vi "Date time format to text sortable.vi"(8 "error in (no error)":errorcluster, 11 "Date time string":string) -> (0 "error out":errorcluster, 3 "New date time string":string)   [LabVIEW 2013]
panel:
  out "PM?":bool
  out "minute":string
  out "hour":string
  out "year":string
  out "day":string="Day"
  out "month":string
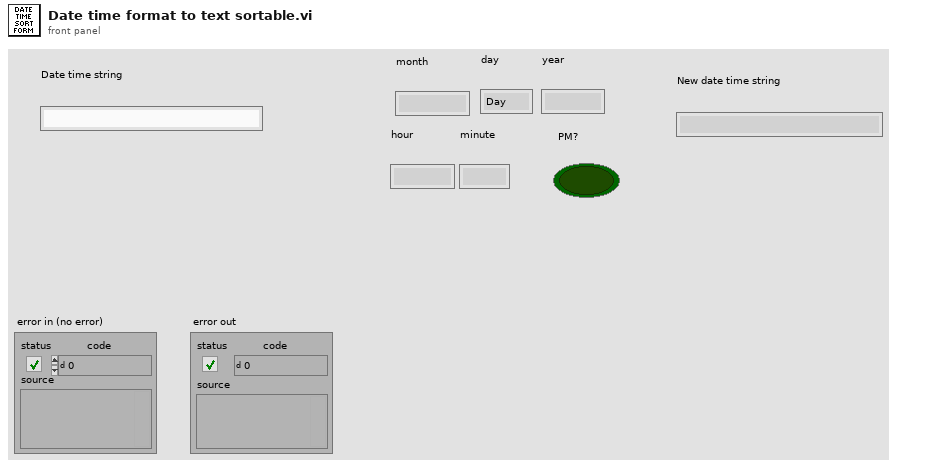
[diagram p1: front panel]
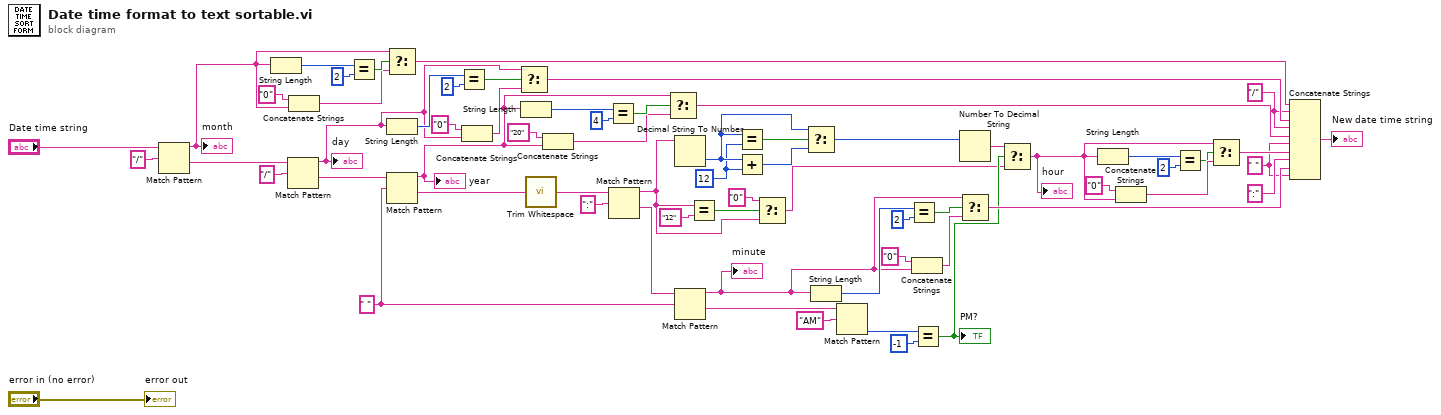
[diagram p0: block diagram]
diagram:
  w10 = 12 ("y")
  w15 = " " ("string")
  w37 = "/" ("string")
  w59 = " " ("regular expression")
  n1 = Match Pattern(string="Date time string", regular expression="/") -> (before substring=w48:string, after substring=w64:string)  [unwired: 1 in, 2 out]
  "month" <- w48
  n2 = String Length(string=w48) -> (length=w51:i32)
  n3 = Match Pattern(string=w64, regular expression="/") -> (before substring=w39:string, after substring=w62:string)  [unwired: 1 in, 2 out]
  "day" <- w39
  n4 = Concatenate Strings("0" ("string"), w48) -> (w46:string)
  n5 = Equal?(x=w51, y=2) -> (x = y?=w49:bool)
  n6 = Select(t=w48, s=w49, f=w46) -> (s? t:f=w45:string)
  n7 = String Length(string=w39) -> (length=w40:i32)
  n8 = Match Pattern(string=w62, regular expression=w59) -> (before substring=w31:string, after substring=w54:string)  [unwired: 1 in, 2 out]
  "year" <- w31
  n9 = Equal?(x=w40, y=2) -> (x = y?=w42:bool)
  n10 = Concatenate Strings("0" ("string"), w39) -> (w44:string)
  n11 = Select(t=w39, s=w42, f=w44) -> (s? t:f=w38:string)
  n12 = String Length(string=w31) -> (length=w36:i32)
  n13 = call <vilib>:"Trim Whitespace.vi"("string"=w54) -> ("trimmed string"=w53:string)  [unwired: 1 in]
  n14 = Concatenate Strings("20" ("string"), w31) -> (w32:string)
  n15 = Equal?(x=w36, y=4) -> (x = y?=w34:bool)
  n16 = Match Pattern(string=w53, regular expression=":") -> (before substring=w2:string, after substring=w60:string)  [unwired: 1 in, 2 out]
  n17 = Select(t=w31, s=w34, f=w32) -> (s? t:f=w30:string)
  n18 = Decimal String To Number(string=w2) -> (number=w11:i32)  [unwired: 2 in, 1 out]
  n19 = Match Pattern(string=w60, regular expression=w59) -> (before substring=w17:string, after substring=w58:string)  [unwired: 1 in, 2 out]
  "minute" <- w17
  n20 = Equal?(x=w2, y="12") -> (x = y?=w4:bool)
  n21 = Equal?(x=w11, y=w10) -> (x = y?=w12:bool)
  n22 = Add(x=w11, y=w10) -> (x+y=w9:i32)
  n23 = Select(t="0", s=w4, f=w2) -> (s? t:f=w1:string)
  n24 = Select(t=w11, s=w12, f=w9) -> (s? t:f=w8:i32)
  n25 = String Length(string=w17) -> (length=w22:i32)
  n26 = Match Pattern(string=w58, regular expression="AM") -> (offset past match=w56:i32)  [unwired: 1 in, 3 out]
  n27 = Equal?(x=w22, y=2) -> (x = y?=w20:bool)
  n28 = Concatenate Strings("0" ("string"), w17) -> (w18:string)
  n29 = Equal?(x=w56, y=-1) -> (x = y?=w13:bool)
  "PM?" <- w13
  n30 = Number To Decimal String(number=w8) -> (decimal integer string=w7:string)  [unwired: 1 in]
  n31 = Select(t=w17, s=w20, f=w18) -> (s? t:f=w16:string)
  n32 = Select(t=w7, s=w13, f=w1) -> (s? t:f=w6:string)
  "hour" <- w6
  n33 = String Length(string=w6) -> (length=w25:i32)
  n34 = Concatenate Strings("0" ("string"), w6) -> (w29:string)
  n35 = Equal?(x=w25, y=2) -> (x = y?=w27:bool)
  n36 = Select(t=w6, s=w27, f=w29) -> (s? t:f=w24:string)
  n37 = Concatenate Strings(w45, w37, w38, w37, w30, w15, w24, ":" ("string"), w16, w15) -> (→"New date time string":string)
  "error out" <- "error in (no error)"
